vi "Connor Heng Prime.vi"() -> ()   [LabVIEW 2012]
panel:
  out "is not prime":bool
  in  "Numeric Control":dbl
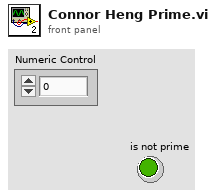
[diagram p1: front panel]
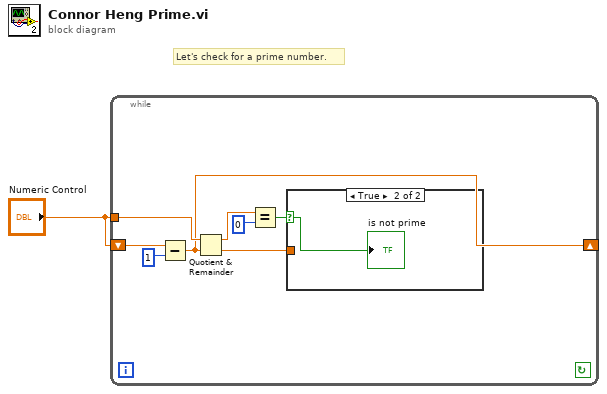
[diagram p0: block diagram]
diagram:
  # "Let's check for a prime number."
  n1 = while {
    shift-right: [w2] -> _
    shift-left: "Numeric Control" -> [w7]
    tunnel: "Numeric Control" -> [w8]
    stop <- _ continue-if-true
    n2 = Subtract(x=w7, y=1) -> (x-y=w2:dbl)
    n3 = Quotient & Remainder(x=w8, y=w2) -> (x-y*floor(x/y)=w3:dbl, floor(x/y)=w6:dbl)
    n4 = Equal?(x=w3, y=0) -> (x = y?=w4:bool)
    n5 = case shown="True" w4 {
      selector: w4 -> [_ w10]
      tunnel: w6 -> [_ _]
      frame False {
      }
      frame True {
        "is not prime" <- w10
      }
    }
  }
